vi "Demag. FINAL.vi"(3 "pomer":dbl, 4 "error in (no error) FUN GEN":errorcluster, 5 "VISA resource name FUN GEN":refnum<visa-resource-name>) -> (0 "error out FUN GEN":errorcluster, 1 "Array":dbl[](array[numeric]), 2 "VISA resource name out FUN GEN":refnum<visa-resource-name>)   [LabVIEW 2018]
panel:
  in  "Typ priebehu":string(combo)="SIN"
  out "krok":dbl
  out "Result":string
  out "Napatie po":dbl
  out "Numeric":i32
  out "Trvanie":dbl
  out "Max napatie":dbl
  out "Pocet priebehov":dbl=10.0
  in  "Combo Box 2":string(combo)="0"
  out "Elapsed Time (s)":dbl
  out "Slide":dbl(slide) scale=0.0..100.0
  out "Frekvencia":dbl=1.0 caption="Time Target (s)"
  in  "stop":bool
  out "zaciatok":dbl
  in  "Boolean":bool
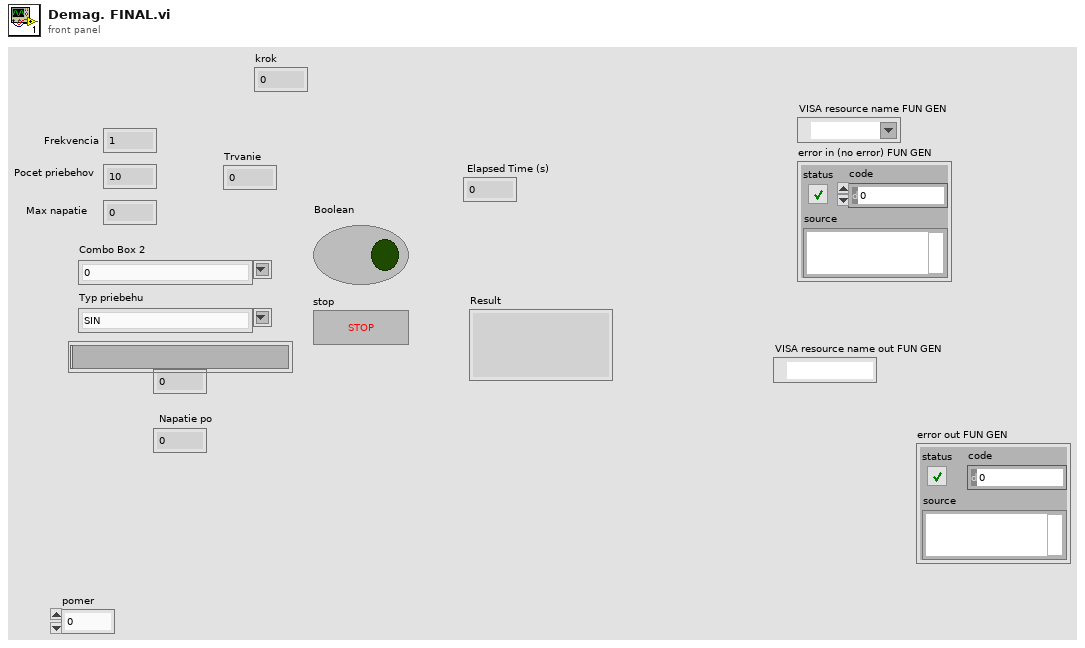
[diagram p1: front panel]
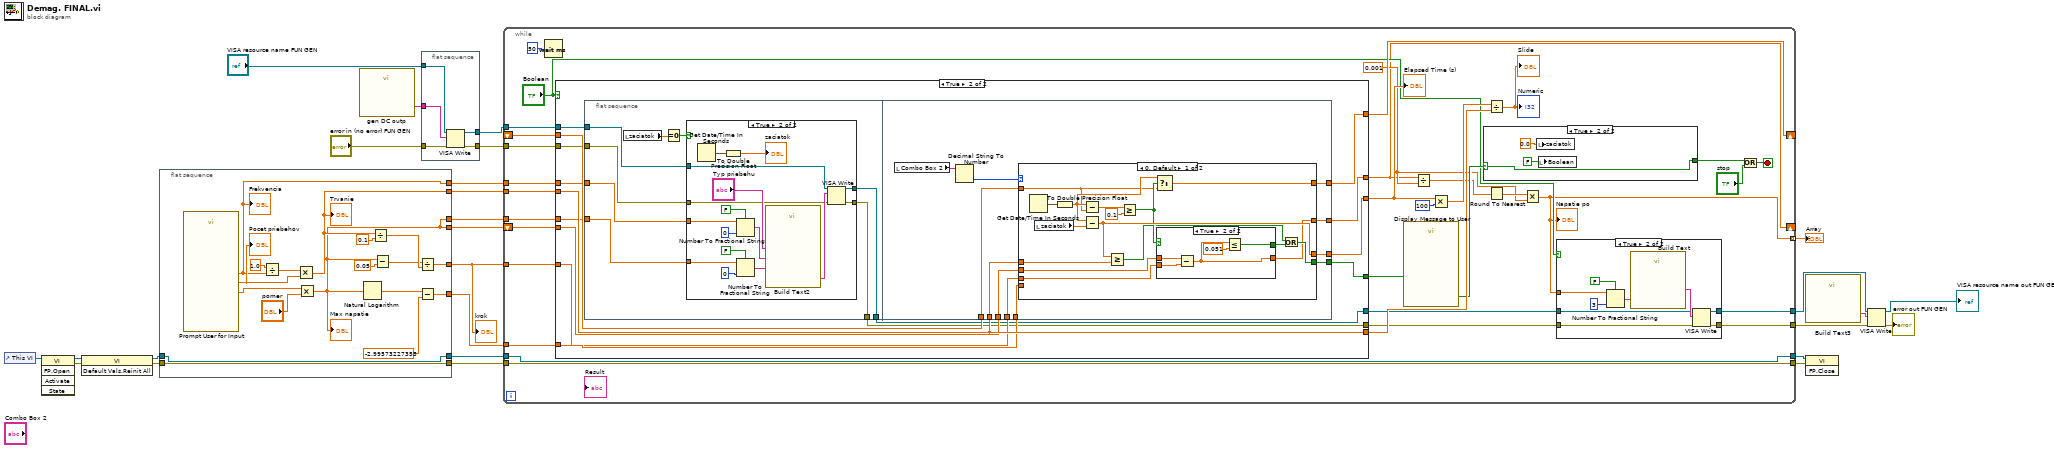
[diagram p0: block diagram]
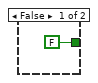
[diagram p3: hidden frame]
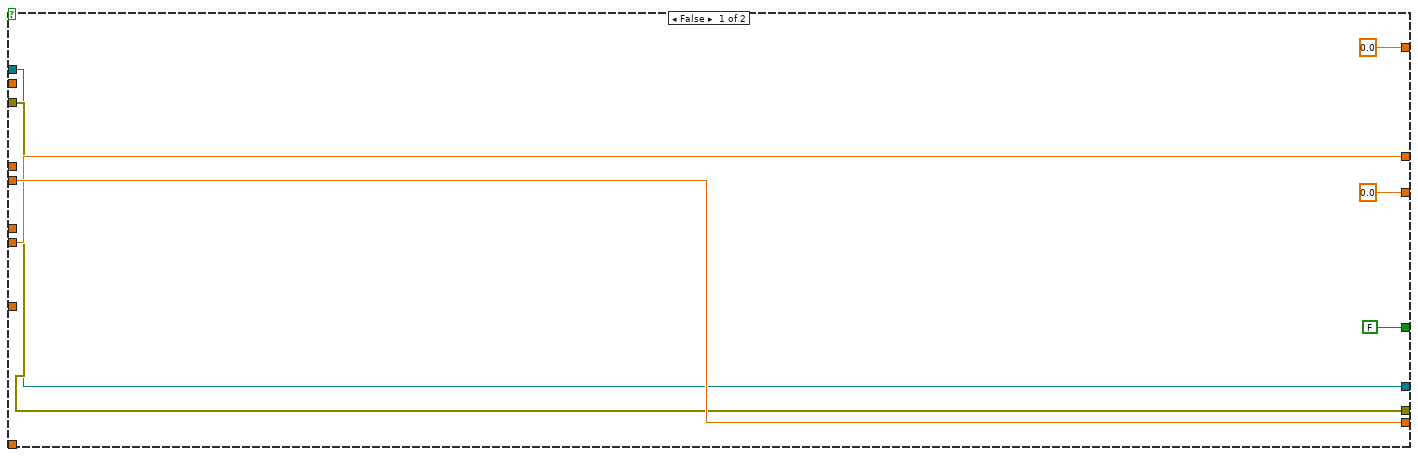
[diagram p4: hidden frame]
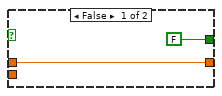
[diagram p6: hidden frame]
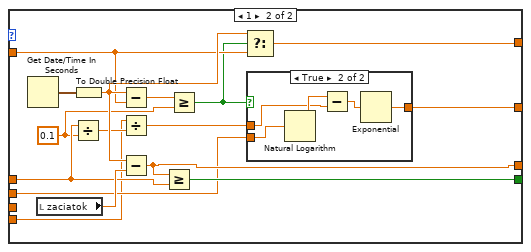
[diagram p7: hidden frame]
diagram:
  n1 = control-ref of="This VI"() -> (w26:refnum<vi>)
  n2 = invoke class="VI" method="FP.Open"(reference=w26) -> (reference out=w25:refnum<vi>, error out=w24:errorcluster)  [unwired: 4 in, 3 out]
  n3 = invoke class="VI" method="Default Vals.Reinit All"(reference=w25, error in=w24) -> (reference out=w20:refnum<vi>, error out=w22:errorcluster)  [unwired: 1 in, 1 out]
  n4 = flat-sequence {
    tunnel: [w44] -> w23
    tunnel: w22 -> [w44]
    tunnel: [w43] -> w21
    tunnel: w20 -> [w43]
    tunnel: [w40] -> w18
    tunnel: [w36] -> w17
    tunnel: [w27] -> w13
    tunnel: [w31] -> w16
    tunnel: [w30] -> w3
    tunnel: [w27] -> w2
    frame #0 {
      n5 = call "Prompt User for Input"() -> ("Max prúd"=w29:dbl, "Pocet priebehov"=w37:dbl, "Frekvencia"=w30:dbl)  [unwired: 15 in, 2 out]
      "Frekvencia" <- w30
      "Pocet priebehov" <- w37
      n6 = Divide(x=1.0, y=w30) -> (x/y=w38:dbl)
      n7 = Multiply(x=w38, y=w37) -> (x*y=w36:dbl)
      "Trvanie" <- w36
      n8 = Multiply(x=w29, y="pomer") -> (x*y=w27:dbl)
      "Max napatie" <- w27
      n9 = Natural Logarithm(1:w27) -> (0:w42:dbl)
      n10 = Divide(x=w36, y=0.1) -> (x/y=w34:dbl)
      n11 = Subtract(x=w27, y=0.05) -> (x-y=w32:dbl)
      n12 = Divide(x=w32, y=w34) -> (x/y=w31:dbl)
      n13 = Subtract(x=w42, y=-2.99573227355) -> (x-y=w40:dbl)
    }
  }
  n14 = call "gen DC outp"() -> ("Result"=w1:string)  [unwired: 14 in, 1 out]
  n15 = flat-sequence {
    tunnel: w1 -> [w49]
    tunnel: "VISA resource name FUN GEN" -> [w48]
    tunnel: "error in (no error) FUN GEN" -> [w47]
    tunnel: [w46] -> w4
    tunnel: [w45] -> w5
    frame #0 {
      n16 = VISA Write(VISA resource name=w48, write buffer=w49, error in (no error)=w47) -> (VISA resource name out=w46:refnum<visa-resource-name>, error out=w45:errorcluster)  [unwired: 1 out]
    }
  }
  n17 = while {
    tunnel: w21 -> [w82]
    tunnel: [w82] -> w12
    tunnel: [w81] -> w11
    tunnel: w23 -> [w81]
    shift-right: [w70] -> _
    shift-left: _ -> [w68]
    shift-right: [w61] -> _
    shift-left: w13 -> [w69]
    tunnel: [w56] -> w19 mode=indexing
    tunnel: w18 -> [w67]
    tunnel: w17 -> [w59]
    tunnel: w16 -> [w60]
    tunnel: [w57] -> w7
    tunnel: [w58] -> w6
    tunnel: w5 -> [w51]
    tunnel: w4 -> [w53]
    tunnel: w3 -> [w55]
    tunnel: w2 -> [w54]
    stop <- w72 stop-if-true
    w62 = 0.001 ("jemnost zaokruhlenia")
    n18 = Wait (ms)(milliseconds to wait=u32 50) -> ()  [unwired: 1 out]
    n19 = case shown="True" "Boolean" {
      tunnel: w59 -> [w102 w118]
      tunnel: [FALSE ("Time has Elapsed") w119] -> w80
      tunnel: [0.0 ("Get Start Time (s)") w113] -> w73
      tunnel: [w102 w118] -> w78
      tunnel: [0.0 ("Get Start Time (s)") w117] -> w70
      tunnel: w68 -> [_ w114]
      tunnel: [w100 w116] -> w61
      tunnel: w69 -> [w100 w115]
      tunnel: w67 -> [_ w112]
      tunnel: w60 -> [_ w111]
      tunnel: w55 -> [_ w110]
      tunnel: w54 -> [_ w109]
      tunnel: w53 -> [w98 w108]
      tunnel: [w98 w107] -> w52
      tunnel: w51 -> [w99 w106]
      tunnel: [w99 w105] -> w50
      frame False {
      }
      frame True {
        n20 = flat-sequence {
          tunnel: w110 -> [w125]
          tunnel: w109 -> [w124]
          tunnel: w108 -> [w123]
          tunnel: [w122] -> w107
          tunnel: w106 -> [w121]
          tunnel: [w120] -> w105
          tunnel: w118 -> [w154]
          tunnel: [w151] -> w119
          tunnel: [w149] -> w117
          tunnel: [w150] -> w116
          tunnel: w115 -> [w153]
          tunnel: w114 -> [w152]
          tunnel: [w148] -> w113
          tunnel: w112 -> [w147]
          tunnel: w111 -> [w146]
          frame #0 {
            n21 = local read "zaciatok"() -> (w127:dbl)
            n22 = Equal To 0?(x=w127) -> (x = 0?=w126:bool)
            n23 = case shown="True" w126 {
              tunnel: w125 -> [_ w136]
              tunnel: w124 -> [_ w135]
              tunnel: w123 -> [w128 w133]
              tunnel: [w128 w132] -> w122
              tunnel: w121 -> [w129 w131]
              tunnel: [w129 w130] -> w120
              frame False {
              }
              frame True {
                n24 = Get Date/Time In Seconds() -> (seconds since 1Jan1904=w145:timestamp)
                n25 = To Double Precision Float(number=w145) -> (double precision float=→"zaciatok":dbl)
                n26 = Number To Fractional String(use system decimal point (T)=FALSE, number=w136, precision (6)=i16 0) -> (F-format string=w142:string)  [unwired: 1 in]
                n27 = Number To Fractional String(use system decimal point (T)=FALSE, number=w135, precision (6)=i16 0) -> (F-format string=w141:string)  [unwired: 1 in]
                n28 = call "Build Text2"("priebeh"="Typ priebehu", "frekv"=w142, "ampl"=w141) -> ("Result"=w134:string)  [unwired: 11 in, 1 out]
                n29 = VISA Write(VISA resource name=w133, write buffer=w134, error in (no error)=w131) -> (VISA resource name out=w132:refnum<visa-resource-name>, error out=w130:errorcluster)  [unwired: 1 out]
              }
            }
          }
          frame #1 {
            n30 = local read "Combo Box 2"() -> (w156:string)
            n31 = Decimal String To Number(string=w156) -> (number=w155:i32)  [unwired: 2 in, 1 out]
            n32 = case shown="0, Default" w155 {
              tunnel: w154 -> [w170 w184]
              tunnel: [w169 w187] -> w148
              tunnel: w153 -> [w163 w186]
              tunnel: w152 -> [w162 w189]
              tunnel: [w161 w193] -> w151
              tunnel: [w160 w185] -> w150
              tunnel: [w159 w192] -> w149
              tunnel: w147 -> [_ w181]
              tunnel: w146 -> [w157 _]
              frame 0, Default {
                n33 = Get Date/Time In Seconds() -> (seconds since 1Jan1904=w172:timestamp)
                n34 = local read "zaciatok"() -> (w171:dbl)
                n35 = To Double Precision Float(number=w172) -> (double precision float=w168:dbl)
                n36 = Subtract(x=w168, y=w162) -> (x-y=w165:dbl)
                n37 = Subtract(x=w168, y=w171) -> (x-y=w169:dbl)
                n38 = Greater Or Equal?(x=w169, y=w170) -> (x >= y?=w164:bool)
                n39 = Greater Or Equal?(x=w165, y=0.1) -> (x >= y?=w166:bool)
                n40 = Select(t=w168, s=w166, f=w162) -> (s? t:f=w159:dbl)
                n41 = case shown="True" w166 {
                  tunnel: [w174 w178] -> w160
                  tunnel: w163 -> [w174 w179]
                  tunnel: [FALSE w176] -> w167
                  tunnel: w157 -> [_ w175]
                  frame False {
                  }
                  frame True {
                    n42 = Subtract(x=w179, y=w175) -> (x-y=w178:dbl)
                    n43 = Less Or Equal?(x=w178, y=0.051) -> (x <= y?=w176:bool)
                  }
                }
                n44 = Or(x=w164, y=w167) -> (x .or. y?=w161:bool)
              }
              frame 1 {
                w183 = 0.1 ("y")
                n45 = Get Date/Time In Seconds() -> (seconds since 1Jan1904=w195:timestamp)
                n46 = local read "zaciatok"() -> (w194:dbl)
                n47 = Divide(x=w184, y=w183) -> (x/y=w182:dbl)
                n48 = To Double Precision Float(number=w195) -> (double precision float=w191:dbl)
                n49 = Subtract(x=w191, y=w189) -> (x-y=w190:dbl)
                n50 = Divide(x=w181, y=w182) -> (x/y=w180:dbl)
                n51 = Subtract(x=w191, y=w194) -> (x-y=w187:dbl)
                n52 = Greater Or Equal?(x=w187, y=w184) -> (x >= y?=w193:bool)
                n53 = Greater Or Equal?(x=w190, y=w183) -> (x >= y?=w188:bool)
                n54 = Select(t=w191, s=w188, f=w189) -> (s? t:f=w192:dbl)
                n55 = case shown="True" w188 {
                  tunnel: w186 -> [w196 w201]
                  tunnel: [w196 w197] -> w185
                  tunnel: w180 -> [_ w199]
                  frame False {
                  }
                  frame True {
                    n56 = Natural Logarithm(1:w201) -> (0:w200:dbl)
                    n57 = Subtract(x=w200, y=w199) -> (x-y=w198:dbl)
                    n58 = Exponential(1:w198) -> (0:w197:dbl)
                  }
                }
              }
            }
          }
        }
      }
    }
    "Elapsed Time (s)" <- w73
    n59 = call "Display Message to User"("Enable"=w80) -> ("OK"=w75:bool)  [unwired: 9 in, 1 out]
    n60 = Divide(x=w61, y=w62) -> (x/y=w64:dbl)
    n61 = Multiply(x=w73, y=100) -> (x*y=w79:dbl)
    n62 = case shown="True" w75 {
      selector: w75 -> [_ w96]
      tunnel: [FALSE w96] -> w74
      frame False {
      }
      frame True {
        n63 = local write "zaciatok"(0.0 ("zaciatok")) -> ()
        n64 = local write "Boolean"(FALSE ("Boolean")) -> ()
      }
    }
    n65 = Divide(x=w79, y=w78) -> (x/y=→"Slide" →"Numeric":dbl)
    n66 = Round To Nearest(number=w64) -> (nearest integer value=w63:dbl)
    n67 = Multiply(x=w63, y=w62) -> (x*y=w56:dbl)
    "Napatie po" <- w56
    n68 = case shown="True" "Boolean" {
      tunnel: w56 -> [_ w93]
      tunnel: w50 -> [w83 w90]
      tunnel: w52 -> [w84 w89]
      tunnel: [w83 w86] -> w58
      tunnel: [w84 w85] -> w57
      frame False {
      }
      frame True {
        n69 = Number To Fractional String(use system decimal point (T)=FALSE, number=w93, precision (6)=i16 3) -> (F-format string=w92:string)  [unwired: 1 in]
        n70 = call "Build Text"("ampl"=w92) -> ("Result"=w91:string)  [unwired: 13 in, 1 out]
        n71 = VISA Write(VISA resource name=w89, write buffer=w91, error in (no error)=w90) -> (VISA resource name out=w85:refnum<visa-resource-name>, error out=w86:errorcluster)  [unwired: 1 out]
      }
    }
    n72 = Or(x=w74, y="stop") -> (x .or. y?=w72:bool)
  }
  "Array" <- w19
  n73 = call "Build Text3"() -> ("Result"=w10:string)  [unwired: 14 in, 1 out]
  n74 = invoke class="VI" method="FP.Close"(reference=w12, error in=w11) -> ()  [unwired: 1 in, 3 out]
  n75 = VISA Write(VISA resource name=w7, write buffer=w10, error in (no error)=w6) -> (VISA resource name out=→"VISA resource name out FUN GEN":refnum<visa-resource-name>, error out=→"error out FUN GEN":errorcluster)  [unwired: 1 out]
  "krok" <- w16
